vi "16TVTI-WriteNeedleValveOutput.vi"(2 "Needle Valve Output (%":dbl min=0.0 max=99.9 format="%.2f", 3 "ITC IO Info":T1={"Com Port"=1, "ISOBUS Address"=1, "GPIB Address"=1, "Communication"=enum."ISOBUS"}) -> (1 "ITC IO Info":T1={"Com Port"=1, "ISOBUS Address"=1, "GPIB Address"=1, "Communication"=enum."ISOBUS"})   [LabVIEW 2018]
doc: "Only relevant to ITC's which control a needle valev."
uses:
  Equipment/Oxford Software/Oxsoft/ITCSUBS.LLB/ITCIO.ctl
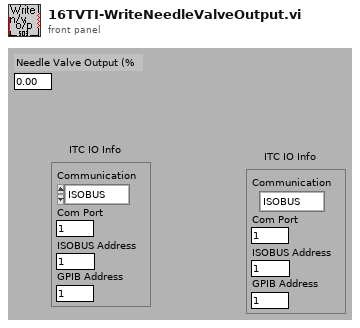
[diagram p1: front panel]
types:
  T1 = typedef "ITCIO.ctl" = cluster{"Com Port":i32, "ISOBUS Address":i32, "GPIB Address":i16, "Communication":enum16{"RS232", "ISOBUS", "GPIB", "Gateway"}}
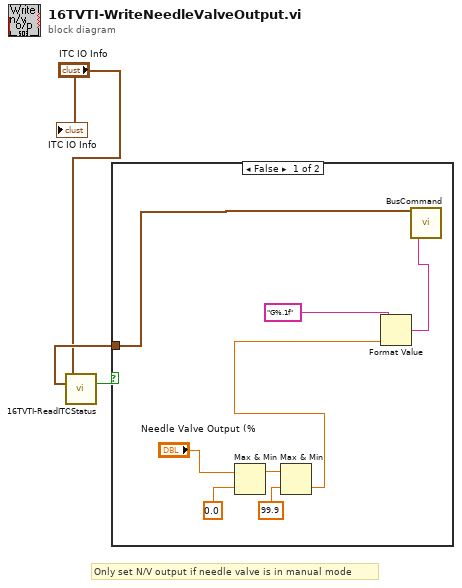
[diagram p0: block diagram]
diagram:
  # "Only set N/V output if needle valve is in manual mode"
  n1 = call "16TVTI-ReadITCStatus.vi"("ITC IO Info"="ITC IO Info") -> ("ITC IO Info"=w3:T1, "Auto Needle Valve"=w1:bool)  [unwired: 4 in, 9 out]
  n2 = case shown="False" w1 {
    tunnel: w3 -> [w4 _]
    frame False {
      n3 = Max & Min(x="Needle Valve Output (%", y=0.0) -> (max(x,y)=w7:dbl)  [unwired: 1 out]
      n4 = Max & Min(x=w7, y=99.9) -> (min(x,y)=w10:dbl)  [unwired: 1 out]
      n5 = Format Value(format string="G%.1f", value (0)=w10) -> (output string=w11:string)  [unwired: 1 in]
      n6 = call "BusCommand.vi"("Command"=w11, "Instrument address (in)"=w4) -> ()  [unwired: 2 out]
    }
    frame True {
    }
  }
  "ITC IO Info" <- "ITC IO Info"
